vi "FGV_AOL Calibration.vi"(7 "Input includes FOV sizes line? (T)":bool=TRUE, 8 "error in (no error)":errorcluster, 9 "Function":T1=enum."Read", 10 "Calibration Data in":dbl[][](array[numeric])=[[-1.0, 148.1, 179.3, 262.9], [-0.8, 118.0, 140.7, 217.8], [-0.6, 90.0, 106.7, 183.1], [-0.4, 59.7, 68.6, 132.8], [-0.2, 27.9, 33.1, 74.0], [0.0, 0.0, 0.0, 0.0], [0.2, -32.0, -50.0, -50.2], [0.4, -65.7, -90.6, -118.9], [0.6, -98.2, -135.6, -196.7], [0.8, -131.7, -182.8, -291.7], [1.0, -168.7, -223.8, -376.0]]) -> (0 "error out":errorcluster, 2 "Calibration Data":dbl[][](array[numeric]), 3 "FOV values":dbl[](array[numeric]))   [LabVIEW 2013]
uses:
  Typedefs/Functional global standard states.ctl
  Typedefs/Read Write Enum.ctl
  Typedefs/Which path.ctl
  gl_Calibration globals.vi
  Program Files (x86)/National Instruments/LabVIEW 2013/user.lib/My Palettes.lib/Files & paths/Spreadsheet/Read From Spreadsheet File (DBL)-Mod.vi
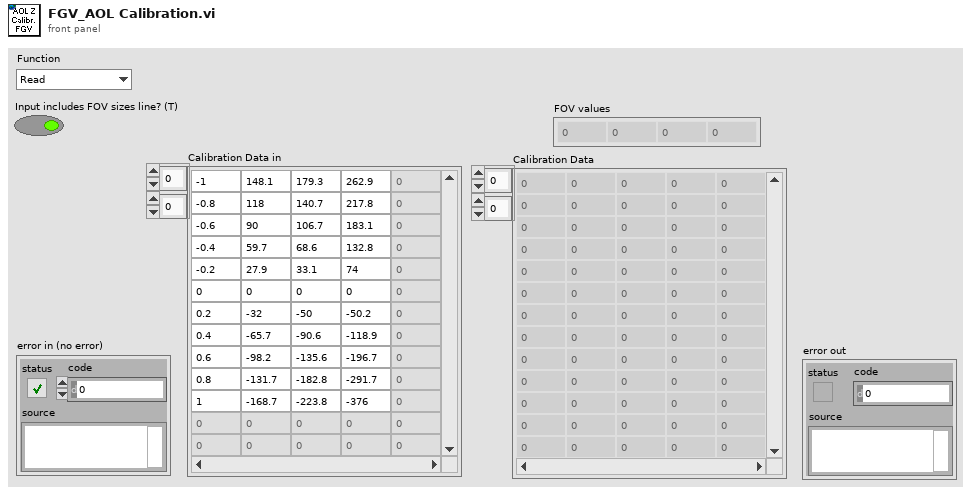
[diagram p1: front panel]
types:
  T1 = typedef "Functional global standard states.ctl" = enum16{"Initialise", "Read", "Write", "Load", "Save", "Clear"}
  T2 = typedef "Which path.ctl" = enum16{"Configuration Files", "Calibration Files", "Images", "Setup.ini", "Loaded User profile.ini", "User's-Previous session.ini", "New user profile.ini", "Selected User profile.ini", "User profiles folder", "Power meter scaling.txt", "FOV Cal.ini"}
  T3 = typedef "Read Write Enum.ctl" = enum16{"Read", "Write"}
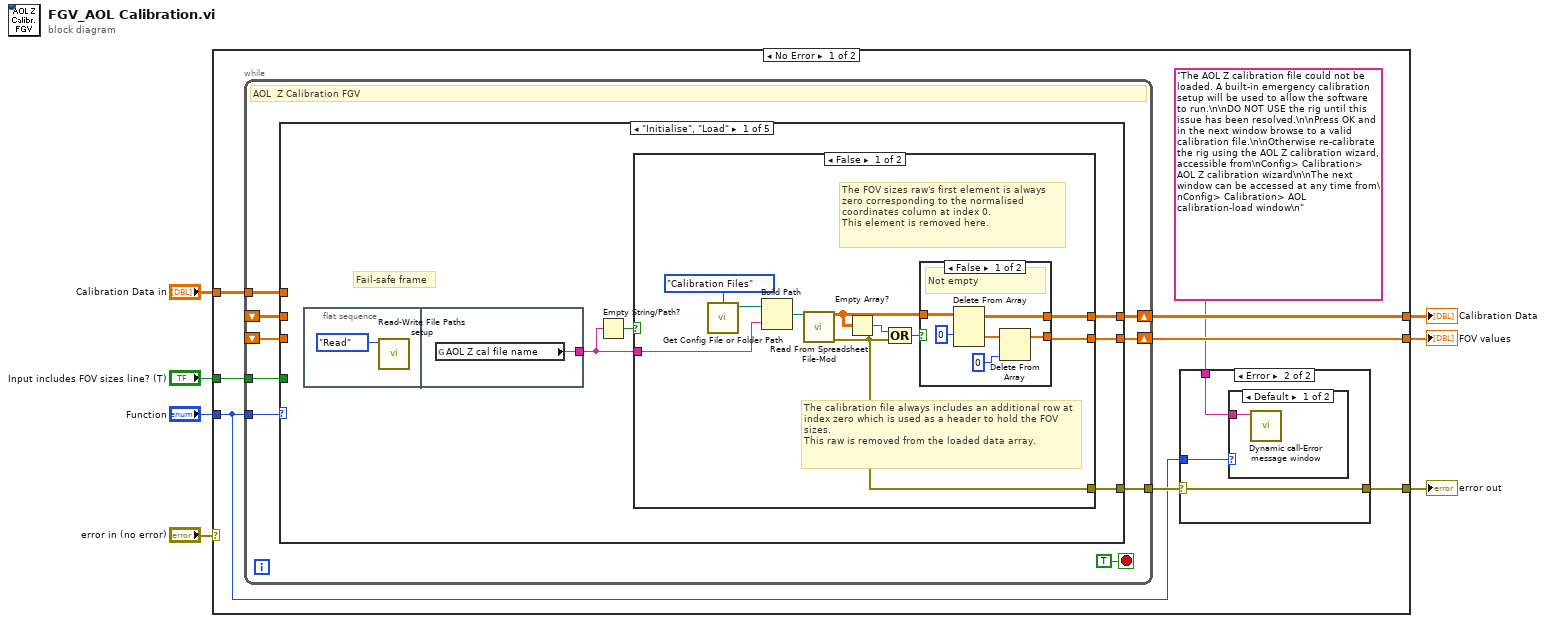
[diagram p0: block diagram]
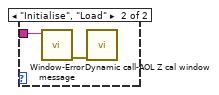
[diagram p3: hidden frame]
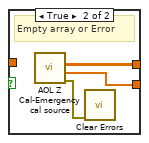
[diagram p4: hidden frame]
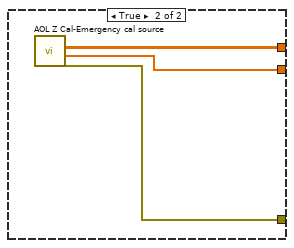
[diagram p5: hidden frame]
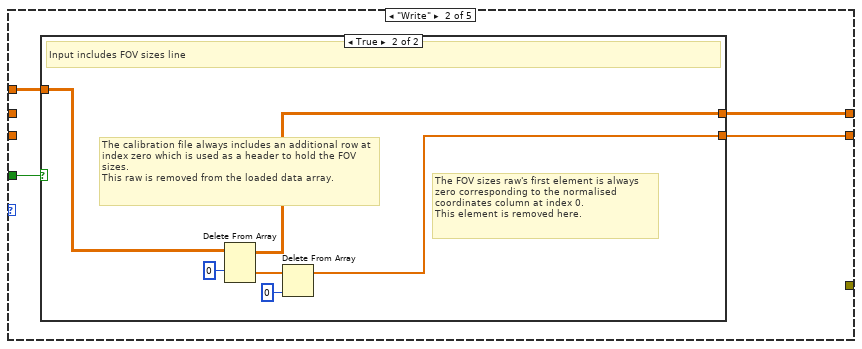
[diagram p6: hidden frame]
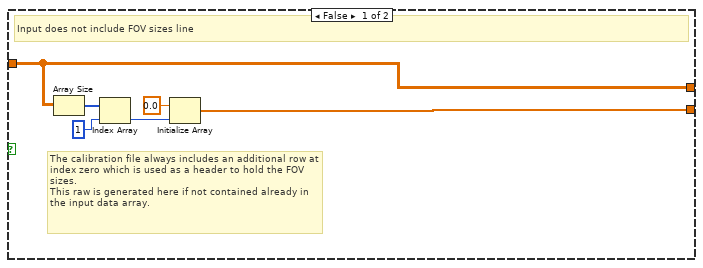
[diagram p7: hidden frame]
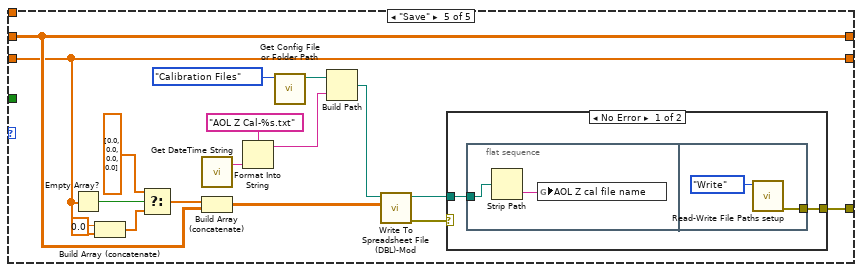
[diagram p10: hidden frame]
diagram:
  n1 = case shown="No Error" "error in (no error)" {
    selector: "error in (no error)" -> [_ w103]
    tunnel: [w10 w103] -> w1
    tunnel: "Function" -> [w8 _]
    tunnel: "Calibration Data in" -> [w15 _]
    tunnel: "Input includes FOV sizes line? (T)" -> [w14 _]
    tunnel: [w13 _] -> w4
    tunnel: [w12 _] -> w3
    frame No Error {
      n2 = while {
        tunnel: w8 -> [w31]
        tunnel: w15 -> [w29]
        tunnel: w14 -> [w28]
        shift-right: [w27] -> w13
        shift-left: _ -> [w26]
        shift-right: [w25] -> w12
        shift-left: _ -> [w24]
        tunnel: [w23] -> w11
        stop <- TRUE stop-if-true
        # "AOL  Z Calibration FGV"
        n3 = case shown="\"Initialise\", \"Load\"" w31 {
          tunnel: [w32 _ _ _ w86] -> w23
          tunnel: w29 -> [_ w64 _ _ _]
          tunnel: w28 -> [_ w62 _ _ _]
          tunnel: [w36 w63 _ w78 w87] -> w27
          tunnel: w26 -> [_ _ _ w78 w87]
          tunnel: [w35 w61 _ w77 w85] -> w25
          tunnel: w24 -> [_ _ _ w77 w85]
          frame "Initialise", "Load" {
            # "Fail-safe frame"
            n4 = flat-sequence {
              tunnel: [w60] -> w34
              frame #0 {
                n5 = call "Read-Write File Paths setup.vi"("Function"=Read_Write_Enum."Read") -> ()  [unwired: 10 in, 1 out]
              }
              frame #1 {
                n6 = global read "gl_Calibration globals.vi" "AOL Z cal file name"() -> (w60:string)
              }
            }
            n7 = Empty String/Path?(string/path=w34) -> (empty?=w33:bool)
            n8 = case shown="False" w33 {
              tunnel: [w44 w58] -> w36
              tunnel: [w43 w57] -> w35
              tunnel: w34 -> [w42 _]
              tunnel: [w38 w56] -> w32
              frame False {
                # "The FOV sizes raw's first element is always zero corresponding to the normalised coordinates column at index 0.\nThis element is removed here."
                # "The calibration file always includes an additional row at index zero which is used as a header to hold the FOV sizes.\nThis raw is removed from the loaded data array."
                n9 = call "Get Config File or Folder Path.vi"("Which file or folder?"=Which_path."Calibration Files" ("Which path?")) -> ("File Path"=w45:path)  [unwired: 8 in, 2 out]
                n10 = Build Path(base path=w45, name or relative path=w42) -> (appended path=w41:path)
                n11 = call-poly "Read From Spreadsheet File-Mod.vi"("file path (dialog if empty)"=w41) -> ("all rows"=w37:dbl[][], "error out"=w38:errorcluster)  [unwired: 9 in, 4 out]
                n12 = Empty Array?(array=w37) -> (empty?=w40:bool)
                n13 = Compound Arithmetic op=OR(w40, w38) -> (w39:bool)
                n14 = case shown="False" w39 {
                  tunnel: w37 -> [w52 _]
                  tunnel: [w48 w55] -> w44
                  tunnel: [w47 w54] -> w43
                  frame False {
                    # "Not empty"
                    n15 = Delete From Array(array=w52, index (row)=0) -> (deleted portion=w50:dbl[], array with subset deleted=w48:dbl[][])  [unwired: 2 in]
                    n16 = Delete From Array(array=w50, index=0) -> (array with subset deleted=w47:dbl[])  [unwired: 1 in, 1 out]
                  }
                  frame True {
                    # "Empty array or Error"
                    n17 = call "AOL Z Cal-Emergency cal source.vi"() -> ("error out"=w53:errorcluster, "FOV Sizes"=w54:dbl[], "Calibration Data"=w55:dbl[][])  [unwired: 9 in]
                    n18 = call <vilib>:"Clear Errors.vi"("error in (no error)"=w53) -> ()  [unwired: 6 in, 1 out]
                  }
                }
              }
              frame True {
                n19 = call "AOL Z Cal-Emergency cal source.vi"() -> ("error out"=w56:errorcluster, "FOV Sizes"=w57:dbl[], "Calibration Data"=w58:dbl[][])  [unwired: 9 in]
              }
            }
          }
          frame "Write" {
            n20 = case shown="True" w62 {
              tunnel: [w70 w71] -> w63
              tunnel: w64 -> [w70 w72]
              tunnel: [w65 w73] -> w61
              frame False {
                # "The calibration file always includes an additional row at index zero which is used as a header to hold the FOV sizes.\nThis raw is generated here if not contained already in the input data array."
                # "Input does not include FOV sizes line"
                n21 = Array Size(array=w70) -> (size(s)=w69:i32[])
                n22 = Index Array(array=w69, index=1) -> (element=w67:i32)
                n23 = Initialize Array(0.0 ("element"), w67) -> (w65:dbl[])
              }
              frame True {
                # "The FOV sizes raw's first element is always zero corresponding to the normalised coordinates column at index 0.\nThis element is removed here."
                # "The calibration file always includes an additional row at index zero which is used as a header to hold the FOV sizes.\nThis raw is removed from the loaded data array."
                # "Input includes FOV sizes line"
                n24 = Delete From Array(array=w72, index (row)=0) -> (deleted portion=w75:dbl[], array with subset deleted=w71:dbl[][])  [unwired: 2 in]
                n25 = Delete From Array(array=w75, index=0) -> (array with subset deleted=w73:dbl[])  [unwired: 1 in, 1 out]
              }
            }
          }
          frame "Clear" {
          }
          frame "Read", Default {
          }
          frame "Save" {
            n26 = Empty Array?(array=w85) -> (empty?=w90:bool)
            n27 = Build Array (concatenate)(0.0, w85) -> (w84:dbl[])
            n28 = Select(t=dbl[] [0.0, 0.0, 0.0, 0.0], s=w90, f=w84) -> (s? t:f=w88:dbl[])
            n29 = call "Get DateTime String.vi"() -> ("date/time string"=w94:string)  [unwired: 10 in, 1 out]
            n30 = Build Array (concatenate)(w88, w87) -> (w81:dbl[][])
            n31 = Format Into String(format string="AOL Z Cal-%s.txt", w94) -> (resulting string=w93:string)  [unwired: 2 in, 1 out]
            n32 = call "Get Config File or Folder Path.vi"("Which file or folder?"=Which_path."Calibration Files" ("Which path?")) -> ("File Path"=w91:path)  [unwired: 8 in, 2 out]
            n33 = Build Path(base path=w91, name or relative path=w93) -> (appended path=w82:path)
            n34 = call "Write To Spreadsheet File (DBL)-Mod.vi"("2D data"=w81, "file path (dialog if empty)"=w82) -> ("error out"=w80:errorcluster, "new file path (Not A Path if cancelled)"=w79:path)  [unwired: 8 in]
            n35 = case shown="No Error" w80 {
              selector: w80 -> [_ w102]
              tunnel: [w96 w102] -> w86
              tunnel: w79 -> [w97 _]
              frame No Error {
                n36 = flat-sequence {
                  tunnel: w97 -> [w99]
                  tunnel: [w100] -> w96
                  frame #0 {
                    n37 = Strip Path(path=w99) -> (name=w98:string)  [unwired: 1 out]
                    n38 = global write "gl_Calibration globals.vi" "AOL Z cal file name"(w98) -> ()
                  }
                  frame #1 {
                    n39 = call "Read-Write File Paths setup.vi"("Function"=Read_Write_Enum."Write") -> ("error out"=w100:errorcluster)  [unwired: 10 in]
                  }
                }
              }
              frame Error {
              }
            }
          }
        }
      }
      n40 = case shown="Error" w11 {
        selector: w11 -> [w16 w19]
        tunnel: [w16 w19] -> w10
        tunnel: "The AOL Z calibration file could not be loaded. A built-in emergency calibration setup will be used to allow the software to run.\n\nDO NOT USE the rig until this issue has been resolved.\n\nPress OK and in the next window browse to a valid calibration file.\n\nOtherwise re-calibrate the rig using the AOL Z calibration wizard, accessible from\nConfig> Calibration> AOL Z calibration wizard\n\nThe next window can be accessed at any time from\nConfig> Calibration> AOL calibration-load window\n" ("Error Message") -> [_ w17]
        tunnel: w8 -> [_ w18]
        frame No Error {
        }
        frame Error {
          n41 = case shown="Default" w18 {
            tunnel: w17 -> [w20 w22]
            frame Default {
              n42 = call "Dynamic call-Error message window.vi"("Error Message"=w20) -> ()  [unwired: 10 in, 1 out]
            }
            frame "Initialise", "Load" {
              n43 = call "Window-Error message.vi"("Message"=w22) -> ("Error Out (no error)"=w21:errorcluster)  [unwired: 10 in]
              n44 = call "Dynamic call-AOL Z cal window.vi"("error in (no error)"=w21) -> ()  [unwired: 10 in, 1 out]
            }
          }
        }
      }
    }
    frame Error {
    }
  }
  "error out" <- w1
  "Calibration Data" <- w4
  "FOV values" <- w3
